vi "Get UI Details.vi"() -> ()   [LabVIEW 2021, in "Stepped Frequency Sweep_Audio DAC.lvlib"]
uses:
  Stepped Frequency Sweep_Audio DAC.lvlib
  <vilib>/Plug-In SDKs/Measurements/Helpers/TypeDefs/User Interface Information.ctl
  <vilib>/Plug-In SDKs/Measurements/NI Measurement Plug-In SDK.lvlib
panel:
  out "error out":errorcluster
  in  "error in":errorcluster
  out "user interface details":T1[](array[typedef])
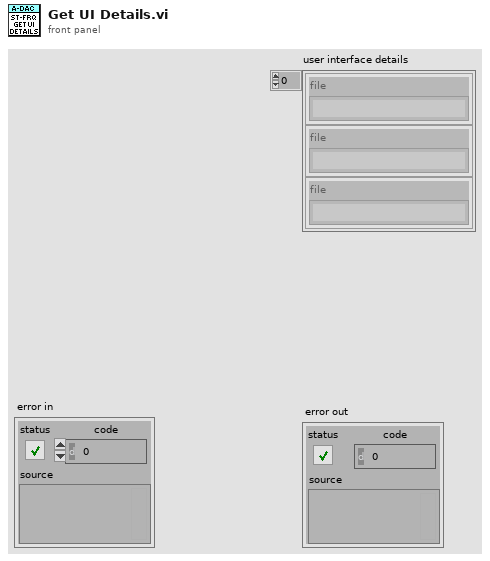
[diagram p1: front panel]
types:
  T1 = typedef "NI Measurement Plug-In SDK.lvlib/User Interface Information.ctl" = cluster{"file":string}
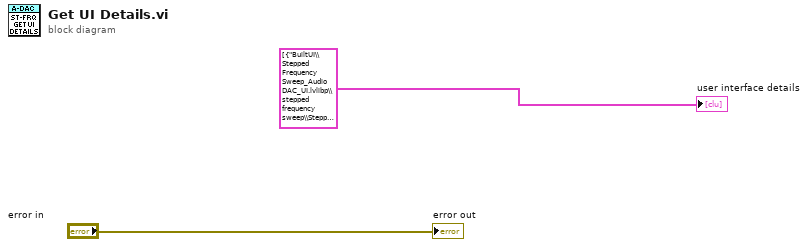
[diagram p0: block diagram]
diagram:
  "user interface details" <- T1[] [{"file"="BuiltUI\\Stepped Frequency Sweep_Audio DAC_UI.lvlibp\\stepped frequency sweep\\Stepped Frequency Sweep_Audio DAC\\Measurement UI.vi"}] ("appended array")
  "error out" <- "error in"
